vi "CAN Initialize.vi"(6 "Interrupt":u16, 7 "IOPort":u32, 8 "error in (no error)":errorcluster caption="错误输入（无错误）", 9 "HwType":u8, 10 "Btr0Btr1":u16, 11 "Channel":u8) -> (0 "error out":errorcluster caption="错误输出", 3 "function return":u32)   [LabVIEW 2021]
doc: "TPCANStatus __stdcall CAN_Initialize(\n TPCANHandle Channel, \n TPCANBaudrate Btr0Btr1, \n TPCANType HwType = 0,\n DWORD IOPort = 0, \n WORD Interrupt = 0);"
uses:
  PCANBasic.dll
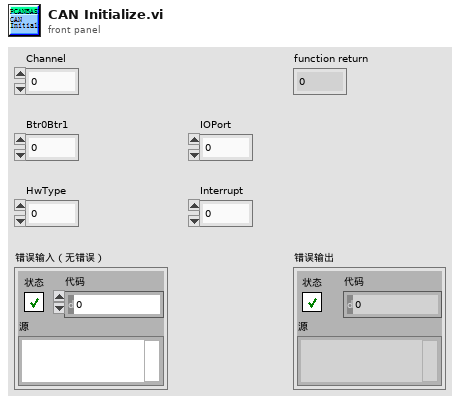
[diagram p1: front panel]
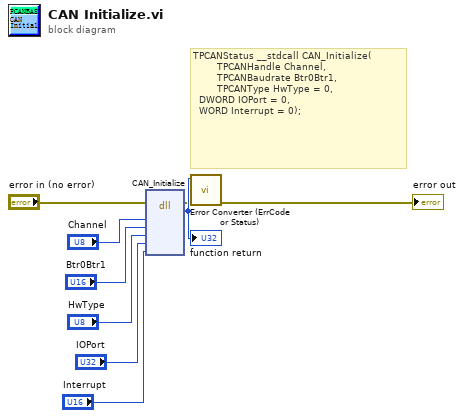
[diagram p0: block diagram]
diagram:
  # "TPCANStatus __stdcall CAN_Initialize(\n        TPCANHandle Channel, \n        TPCANBaudrate Btr0Btr1, \n        TPCANType HwType = 0,\n\t\tDWORD IOPort = 0, \n\t\tWORD Interrupt = 0);"
  n1 = dll-call lib="D:/ON LINE WORK/LabVIEW/PCAN/PCAN 1.6(2021)/PCANBasic.dll" fn="CAN_Initialize"(error in="error in (no error)", "Channel"="Channel", "Btr0Btr1"="Btr0Btr1", "HwType"="HwType", "IOPort"="IOPort", "Interrupt"="Interrupt") -> (error out=w2:errorcluster, "返回类型"=w9:u32)  [unwired: 7 in, 1 out]
  "function return" <- w9
  n2 = call "Error Converter (ErrCode or Status).vi"("error in (no error)"=w2, "error code"=w9) -> ("error out"=→"error out":errorcluster)  [unwired: 9 in]
